vi "Add Data Replay Loop.vi"(8 "error in (no error)":errorcluster, 10 "DataReplay Loop":T2, 11 "Crank Cams Page in":T1 format="%.0x") -> (0 "error out":errorcluster, 3 "Parent Ref out":T1 format="%.0x")   [LabVIEW 2011, in "Engine Sim System Explorer.lvlib"]
uses:
  Engine Sim System Explorer.lvlib
  <vilib>/NI Veristand/Custom Device API/Custom Device Item Ref.ctl
  TypeDefs/DataReplayLoopComp.ctl
  TypeDefs/DataReplayComp.ctl
  Shared/Engine Simulation Global.vi
  <vilib>/NI Veristand/Custom Device API/NI VeriStand - Set Item Property.vi
  <vilib>/NI Veristand/Custom Device API/Set Item Property (Boolean).vi
  <vilib>/Utility/error.llb/Error Cluster From Error Code.vi
  <vilib>/NI Veristand/Custom Device API/NI VeriStand - Add Custom Device Channel.vi
  <vilib>/NI Veristand/Custom Device API/Custom Device API.lvlib
  Engine Simulation Shared.lvlib
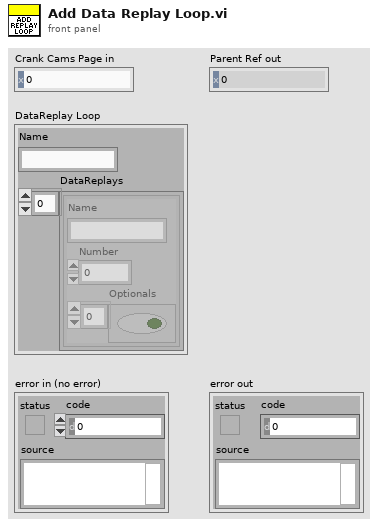
[diagram p1: front panel]
types:
  T1 = typedef "Custom Device API.lvlib/Custom Device Item Ref.ctl" = u64
  T2 = typedef "Engine Sim System Explorer.lvlib/DataReplayLoopComp.ctl" = cluster{"Name":string, "DataReplays":T3[]}
  T3 = typedef "Engine Sim System Explorer.lvlib/DataReplayComp.ctl" = cluster{"Name":string, "Number":i32, "Optionals":bool[]}
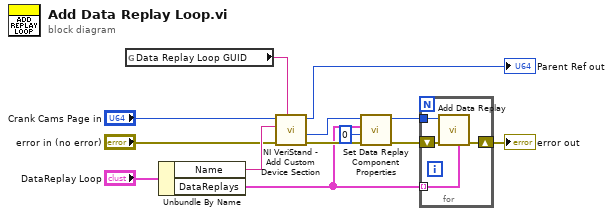
[diagram p0: block diagram]
diagram:
  n1 = global read "Engine Simulation Global.vi" "Data Replay Loop GUID"() -> (w13:string)
  n2 = Unbundle By Name("DataReplay Loop") -> ("Name"=w9:string, "DataReplays"=w2:T3[])
  n3 = call <vilib>:"NI VeriStand - Add Custom Device Section.vi"("GUID (Default Section)"=w13, "error in (no error)"="error in (no error)", "Section Name"=w9, "Parent Ref in"="Crank Cams Page in") -> ("error out"=w10:errorcluster, "Section Ptr"=w4:T1, "Parent Ref out"=→"Parent Ref out":T1)  [unwired: 4 in, 1 out]
  n4 = call "Set Data Replay Component Properties.vi"("error in (no error)"=w10, "Prefix#"=0, "DataReplays"=w2, "Item Ref in"=w4) -> ("error out"=w5:errorcluster, "Item Ref out"=w3:T1)  [unwired: 6 in]
  n5 = for {
    tunnel: w2 -> [w15] mode=indexing
    tunnel: w3 -> [w14]
    shift-right: [w16] -> w11
    shift-left: w5 -> [w17]
    n6 = call "Add Data Replay.vi"("DataReplay"=w15, "error in (no error)"=w17, "Section Ptr"=w14) -> ("error out"=w16:errorcluster)  [unwired: 8 in]
  }
  "error out" <- w11
